vi "myRIO v1.0 Config DI IRQ.vi"(5 "Enable IRQ?":bool, 6 "Edge Count":u32, 7 "IRQ Number":u8, 8 "error in (no error)":errorcluster, 9 "IO IRQ Channels Enum":T1, 10 "IRQ Type":T3, 11 "myRIO FPGA Ref In":T2) -> (0 "error out":errorcluster)   [LabVIEW 2021]
uses:
  <vilib>/myRIO/Common/Instrument Driver Framework/myRIO v1.0/IRQ/typedefs/IRQ Type.ctl
  <vilib>/myRIO/Common/Instrument Driver Framework/Utilities/typedefs/Generic FPGA Reference.ctl
  <vilib>/myRIO/Common/Instrument Driver Framework/myRIO v1.0/IRQ/typedefs/IO IRQ Channels Enum.ctl
  <vilib>/myRIO/Common/Instrument Driver Framework/myRIO v1.0/IRQ/typedefs/DI IRQ FPGA Reference.ctl
  <vilib>/Utility/error.llb/Error Cluster From Error Code.vi
  <vilib>/rvi/errors/niLvFpgaAdjustHostInterfaceError.vi
  <vilib>/rvi/interface/nirviReadWriteControl/nirviReadWriteControl.xnode
  <vilib>/rvi/interface/Simulation/niFpgaSimulationCallBeginRW.vi
  NiFpgaLv.dll
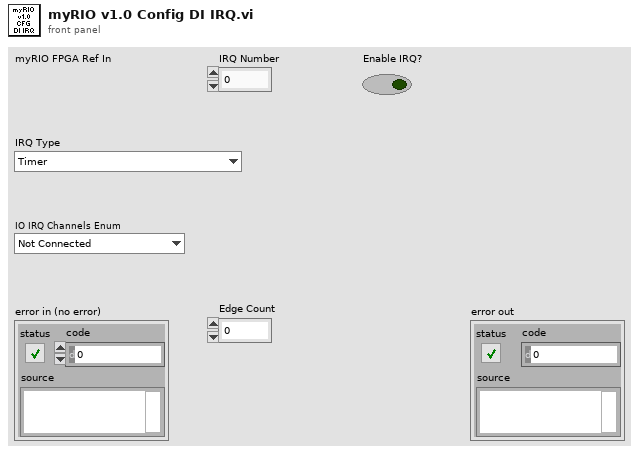
[diagram p1: front panel]
types:
  T1 = typedef "IO IRQ Channels Enum.ctl" = enum16{"Not Connected", "A/AI0 (Interrupt)", "A/AI1 (Interrupt)", "A/DIO0 (Interrupt)", "A/DIO1 (Interrupt)", "A/DIO2 (Interrupt)", "A/DIO3 (Interrupt)", "Button0 (Interrupt)", "B/AI0 (Interrupt)", "B/AI1 (Interrupt)", "B/DIO0 (Interrupt)", "B/DIO1 (Interrupt)", "B/DIO2 (Interrupt)", "B/DIO3 (Interrupt)"}
  T2 = typedef "Generic FPGA Reference.ctl" = refnum<k20>
  T3 = typedef "IRQ Type.ctl" = enum16{"Timer", "Analog falling edge", "Analog rising edge", "Digital falling edge", "Digital rising edge", "Digital edge"}
  T4 = typedef "DI IRQ FPGA Reference.ctl" = refnum<k20>
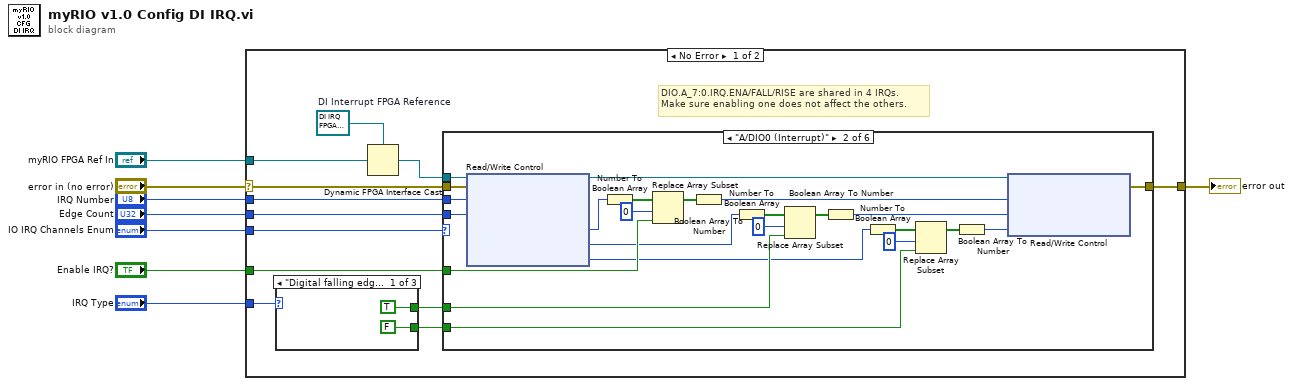
[diagram p0: block diagram]
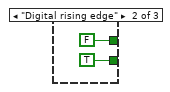
[diagram p2: hidden frame]
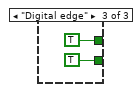
[diagram p3: hidden frame]
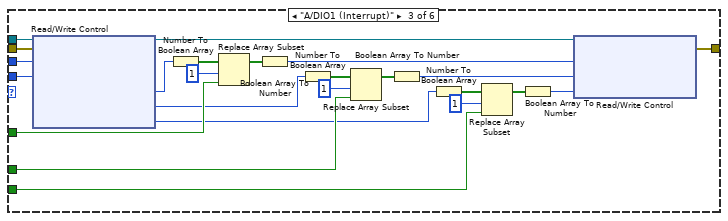
[diagram p5: hidden frame]
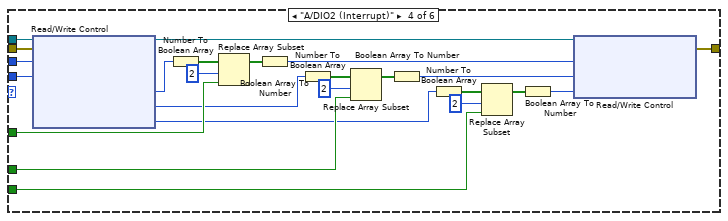
[diagram p6: hidden frame]
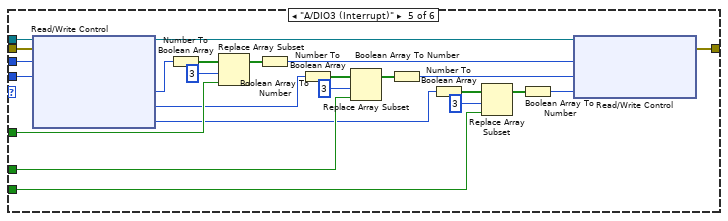
[diagram p7: hidden frame]
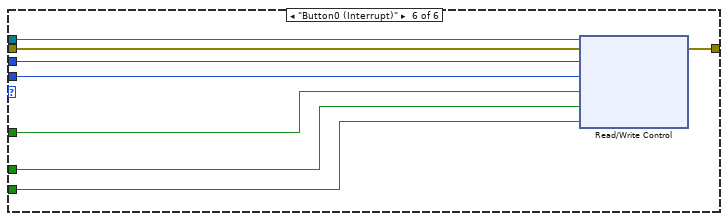
[diagram p8: hidden frame]
diagram:
  n1 = case shown="No Error" "error in (no error)" {
    selector: "error in (no error)" -> [w15 w132]
    tunnel: [w12 w132] -> w8
    tunnel: "IRQ Type" -> [w11 _]
    tunnel: "IRQ Number" -> [w10 _]
    tunnel: "myRIO FPGA Ref In" -> [w20 _]
    tunnel: "IO IRQ Channels Enum" -> [w13 _]
    tunnel: "Edge Count" -> [w14 _]
    tunnel: "Enable IRQ?" -> [w9 _]
    frame No Error {
      w19 = T4 refnum  # DI Interrupt FPGA Reference
      # "DIO.A_7:0.IRQ.ENA/FALL/RISE are shared in 4 IRQs.\nMake sure enabling one does not affect the others."
      n2 = case shown="\"Digital falling edge\", Default" w11 {
        tunnel: [TRUE FALSE TRUE] -> w18
        tunnel: [FALSE TRUE TRUE] -> w17
        frame "Digital falling edge", Default {
        }
        frame "Digital rising edge" {
        }
        frame "Digital edge" {
        }
      }
      n3 = Dynamic FPGA Interface Cast(Session In=w19, Type=w20) -> (Session Out=w16:T4)
      n4 = case shown="\"A/DIO0 (Interrupt)\"" w13 {
        tunnel: w16 -> [_ w35 w59 w87 w111 w131]
        tunnel: w10 -> [_ w33 w57 w85 w109 w129]
        tunnel: w14 -> [_ w32 w56 w84 w108 w128]
        tunnel: w15 -> [w27 w34 w58 w86 w110 w130]
        tunnel: [w27 w36 w60 w80 w104 w124] -> w12
        tunnel: w18 -> [_ w41 w65 w89 w113 w126]
        tunnel: w17 -> [_ w40 w64 w88 w112 w125]
        tunnel: w9 -> [_ w48 w72 w96 w120 w127]
        frame Default {
        }
        frame "A/DIO0 (Interrupt)" {
          n5 = xnode "Read/Write Control"("FPGA VI Reference In"=w35, "error in"=w34, "IRQ.DIO_A_0.NO"=w33, "IRQ.DIO_A_0.CNT"=w32) -> ("FPGA VI Reference Out"=w31:T4, "IRQ.DIO_A_7:0.ENA"=w30:u8, "IRQ.DIO_A_7:0.FALL"=w29:u8, "IRQ.DIO_A_7:0.RISE"=w28:u8)  [unwired: 1 out]
          n6 = Number To Boolean Array(number=w30) -> (Boolean array=w50:bool[])
          n7 = Replace Array Subset(array=w50, new element=w48, index=0) -> (w51:bool[])
          n8 = Boolean Array To Number(Boolean array=w51) -> (number=w39:u8)
          n9 = Number To Boolean Array(number=w29) -> (Boolean array=w46:bool[])
          n10 = Replace Array Subset(array=w46, new element=w41, index=0) -> (w45:bool[])
          n11 = Boolean Array To Number(Boolean array=w45) -> (number=w38:u8)
          n12 = Number To Boolean Array(number=w28) -> (Boolean array=w43:bool[])
          n13 = Replace Array Subset(array=w43, new element=w40, index=0) -> (w44:bool[])
          n14 = Boolean Array To Number(Boolean array=w44) -> (number=w37:u8)
          n15 = xnode "Read/Write Control"("FPGA VI Reference In"=w31, "IRQ.DIO_A_7:0.ENA"=w39, "IRQ.DIO_A_7:0.FALL"=w38, "IRQ.DIO_A_7:0.RISE"=w37) -> ("error out"=w36:errorcluster)  [unwired: 1 in, 1 out]
        }
        frame "A/DIO1 (Interrupt)" {
          n16 = xnode "Read/Write Control"("FPGA VI Reference In"=w59, "error in"=w58, "IRQ.DIO_A_1.NO"=w57, "IRQ.DIO_A_1.CNT"=w56) -> ("FPGA VI Reference Out"=w55:T4, "IRQ.DIO_A_7:0.ENA"=w54:u8, "IRQ.DIO_A_7:0.FALL"=w53:u8, "IRQ.DIO_A_7:0.RISE"=w52:u8)  [unwired: 1 out]
          n17 = Number To Boolean Array(number=w54) -> (Boolean array=w74:bool[])
          n18 = Replace Array Subset(array=w74, new element=w72, index=1) -> (w75:bool[])
          n19 = Boolean Array To Number(Boolean array=w75) -> (number=w63:u8)
          n20 = Number To Boolean Array(number=w53) -> (Boolean array=w70:bool[])
          n21 = Replace Array Subset(array=w70, new element=w65, index=1) -> (w69:bool[])
          n22 = Boolean Array To Number(Boolean array=w69) -> (number=w62:u8)
          n23 = Number To Boolean Array(number=w52) -> (Boolean array=w67:bool[])
          n24 = Replace Array Subset(array=w67, new element=w64, index=1) -> (w68:bool[])
          n25 = Boolean Array To Number(Boolean array=w68) -> (number=w61:u8)
          n26 = xnode "Read/Write Control"("FPGA VI Reference In"=w55, "IRQ.DIO_A_7:0.ENA"=w63, "IRQ.DIO_A_7:0.FALL"=w62, "IRQ.DIO_A_7:0.RISE"=w61) -> ("error out"=w60:errorcluster)  [unwired: 1 in, 1 out]
        }
        frame "A/DIO2 (Interrupt)" {
          n27 = xnode "Read/Write Control"("FPGA VI Reference In"=w87, "error in"=w86, "IRQ.DIO_A_2.NO"=w85, "IRQ.DIO_A_2.CNT"=w84) -> ("FPGA VI Reference Out"=w79:T4, "IRQ.DIO_A_7:0.ENA"=w83:u8, "IRQ.DIO_A_7:0.FALL"=w82:u8, "IRQ.DIO_A_7:0.RISE"=w81:u8)  [unwired: 1 out]
          n28 = Number To Boolean Array(number=w83) -> (Boolean array=w98:bool[])
          n29 = Replace Array Subset(array=w98, new element=w96, index=2) -> (w99:bool[])
          n30 = Boolean Array To Number(Boolean array=w99) -> (number=w78:u8)
          n31 = Number To Boolean Array(number=w82) -> (Boolean array=w94:bool[])
          n32 = Replace Array Subset(array=w94, new element=w89, index=2) -> (w93:bool[])
          n33 = Boolean Array To Number(Boolean array=w93) -> (number=w77:u8)
          n34 = Number To Boolean Array(number=w81) -> (Boolean array=w91:bool[])
          n35 = Replace Array Subset(array=w91, new element=w88, index=2) -> (w92:bool[])
          n36 = Boolean Array To Number(Boolean array=w92) -> (number=w76:u8)
          n37 = xnode "Read/Write Control"("FPGA VI Reference In"=w79, "IRQ.DIO_A_7:0.ENA"=w78, "IRQ.DIO_A_7:0.FALL"=w77, "IRQ.DIO_A_7:0.RISE"=w76) -> ("error out"=w80:errorcluster)  [unwired: 1 in, 1 out]
        }
        frame "A/DIO3 (Interrupt)" {
          n38 = xnode "Read/Write Control"("FPGA VI Reference In"=w111, "error in"=w110, "IRQ.DIO_A_3.NO"=w109, "IRQ.DIO_A_3.CNT"=w108) -> ("FPGA VI Reference Out"=w103:T4, "IRQ.DIO_A_7:0.ENA"=w107:u8, "IRQ.DIO_A_7:0.FALL"=w106:u8, "IRQ.DIO_A_7:0.RISE"=w105:u8)  [unwired: 1 out]
          n39 = Number To Boolean Array(number=w107) -> (Boolean array=w122:bool[])
          n40 = Replace Array Subset(array=w122, new element=w120, index=3) -> (w123:bool[])
          n41 = Boolean Array To Number(Boolean array=w123) -> (number=w102:u8)
          n42 = Number To Boolean Array(number=w106) -> (Boolean array=w118:bool[])
          n43 = Replace Array Subset(array=w118, new element=w113, index=3) -> (w117:bool[])
          n44 = Boolean Array To Number(Boolean array=w117) -> (number=w101:u8)
          n45 = Number To Boolean Array(number=w105) -> (Boolean array=w115:bool[])
          n46 = Replace Array Subset(array=w115, new element=w112, index=3) -> (w116:bool[])
          n47 = Boolean Array To Number(Boolean array=w116) -> (number=w100:u8)
          n48 = xnode "Read/Write Control"("FPGA VI Reference In"=w103, "IRQ.DIO_A_7:0.ENA"=w102, "IRQ.DIO_A_7:0.FALL"=w101, "IRQ.DIO_A_7:0.RISE"=w100) -> ("error out"=w104:errorcluster)  [unwired: 1 in, 1 out]
        }
        frame "Button0 (Interrupt)" {
          n49 = xnode "Read/Write Control"("FPGA VI Reference In"=w131, "error in"=w130, "IRQ.DI_BTN.NO"=w129, "IRQ.DI_BTN.CNT"=w128, "IRQ.DI_BTN.ENA"=w127, "IRQ.DI_BTN.FALL"=w126, "IRQ.DI_BTN.RISE"=w125) -> ("error out"=w124:errorcluster)  [unwired: 1 out]
        }
      }
    }
    frame Error {
    }
  }
  "error out" <- w8
